vi "AutoRun.vi"() -> ()   [LabVIEW 2016]
uses:
  AutoSteps.ctl
  <vilib>/userdefined/High Color/IMAQdx.ctl
  <vilib>/vision/driver/IMAQdx.llb/IMAQdx Acquisition Mode.ctl
  <vilib>/vision/driver/IMAQdx.llb/IMAQdx Buffer Number Mode.ctl
  <vilib>/vision/driver/NI_Vision_Acquisition_Software.lvlib
panel:
  out "Fitted Circle":T1
  out "ListPoints":dbl[][](array[numeric])
  out "CircleY":dbl
  out "CircleX":dbl
  out "Matches":T2(array[cluster])
  out "形状":enum16{"", "圆形", "三角形", "正方形"}(ring)
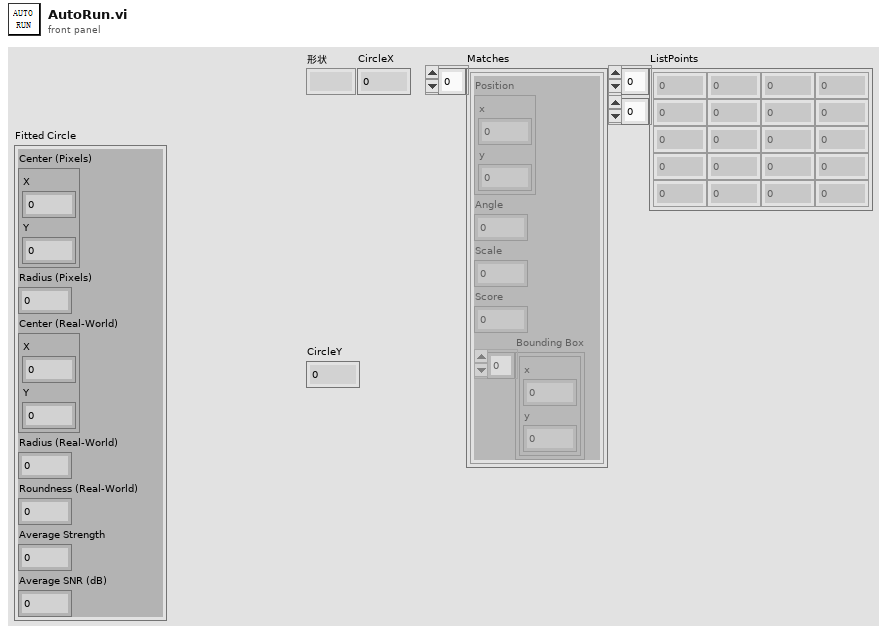
[diagram p1: front panel]
types:
  T1 = cluster{"Center (Pixels)":cluster{"X":sgl, "Y":sgl}, "Radius (Pixels)":dbl, "Center (Real-World)":cluster{"X":sgl, "Y":sgl}, "Radius (Real-World)":dbl, "Roundness (Real-World)":dbl, "Average Strength":dbl, "Average SNR (dB)":dbl}
  T2 = cluster{"Position":cluster{"x":sgl, "y":sgl}, "Angle":sgl, "Scale":sgl, "Score":sgl, "Bounding Box":cluster{"x":sgl, "y":sgl}[]}[]
  T3 = cluster{"Circle":cluster{"CirclePath":path, "Steps":dbl[][], "Points":dbl[][]}, "Trangle":cluster{"TranglePath":path, "Steps":dbl[][], "Points":dbl[][]}, "Square":cluster{"SquarePath":path, "Steps":dbl[][], "Points":dbl[][]}, "Camera":dbl[], "Robot":dbl[]}
  T4 = typedef "AutoSteps.ctl" = enum16{"Nothing", "Initial", "ReadConf", "Wait", "Snap", "ProcePic", "Calculate", "TrancetoPLC", "Error", "Exit"}
  T5 = typedef "IMAQ Image.ctl" = refnum<image>
  T6 = typedef "NI_Vision_Acquisition_Software.lvlib/IMAQdx Acquisition Mode.ctl" = enum32{"One Shot", "Continuous"}
  T7 = typedef "NI_Vision_Acquisition_Software.lvlib/IMAQdx Buffer Number Mode.ctl" = enum32{"Next", "Last", "Buffer Number", "Every", "Last New"}
  T8 = typedef "IMAQdx.ctl" = refnum<k21>
  T9 = cluster{"Position":cluster{"x":sgl, "y":sgl}, "Angle":sgl, "Scale":sgl, "Score":sgl, "Bounding Box":cluster{"x":sgl, "y":sgl}[]}
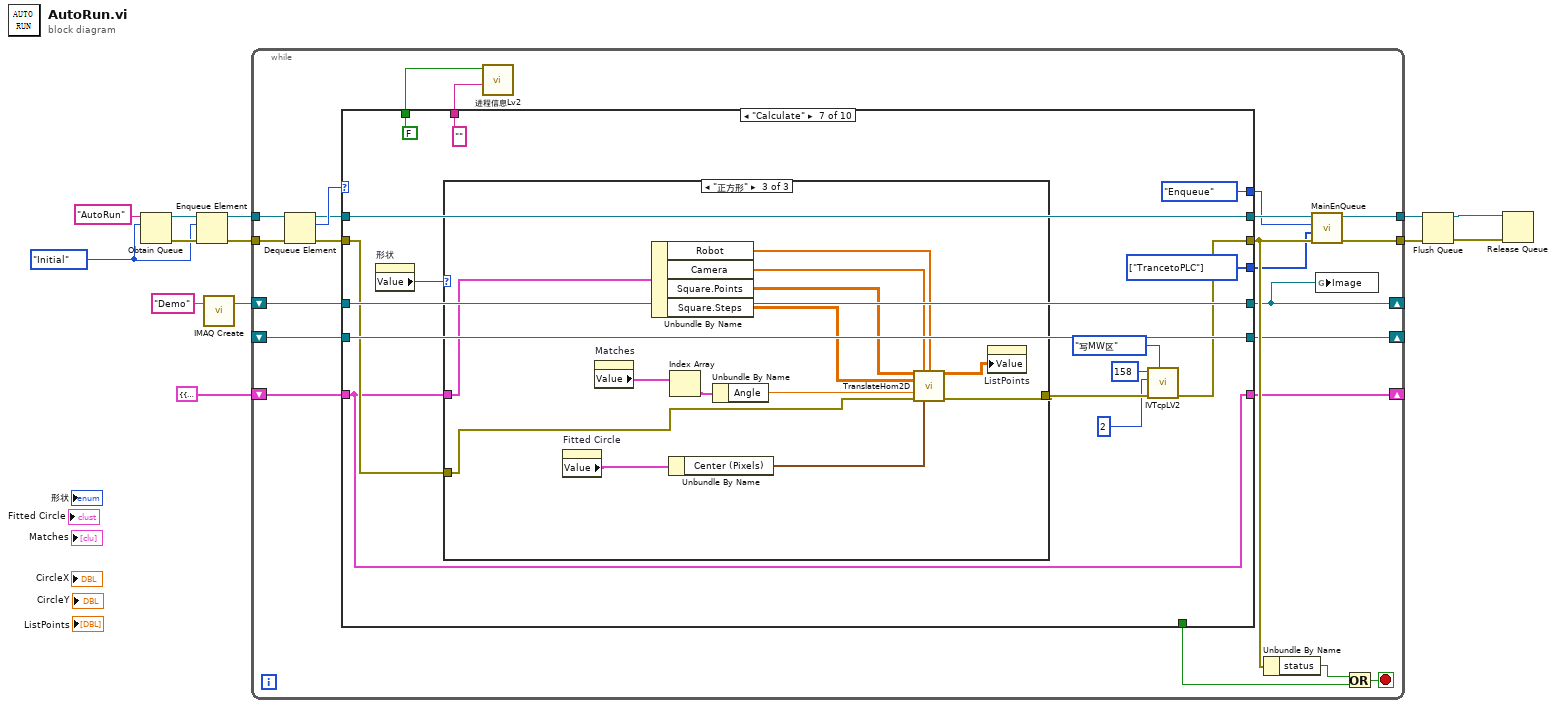
[diagram p0: block diagram]
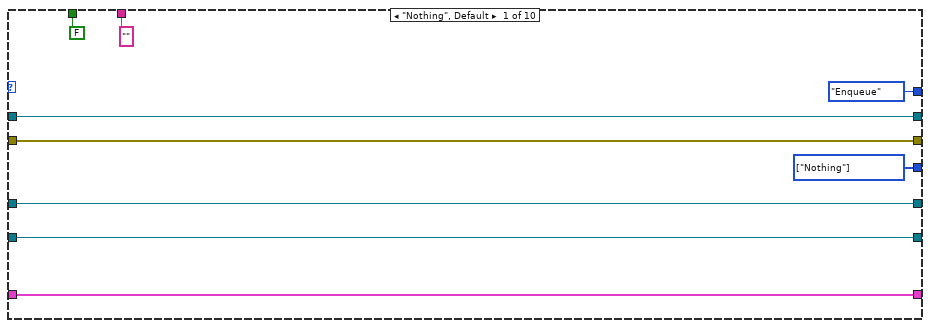
[diagram p2: hidden frame]
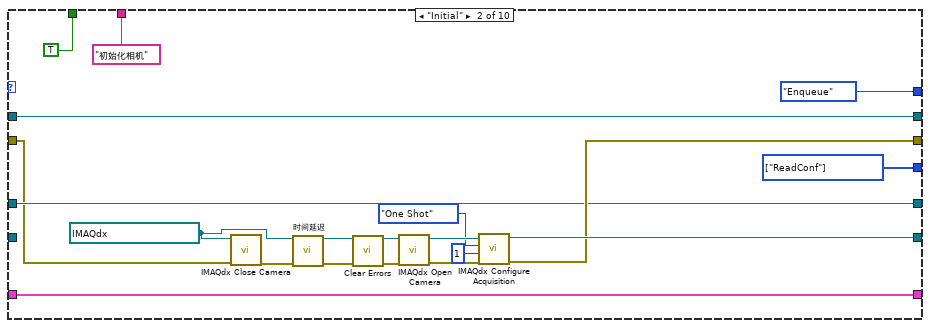
[diagram p3: hidden frame]
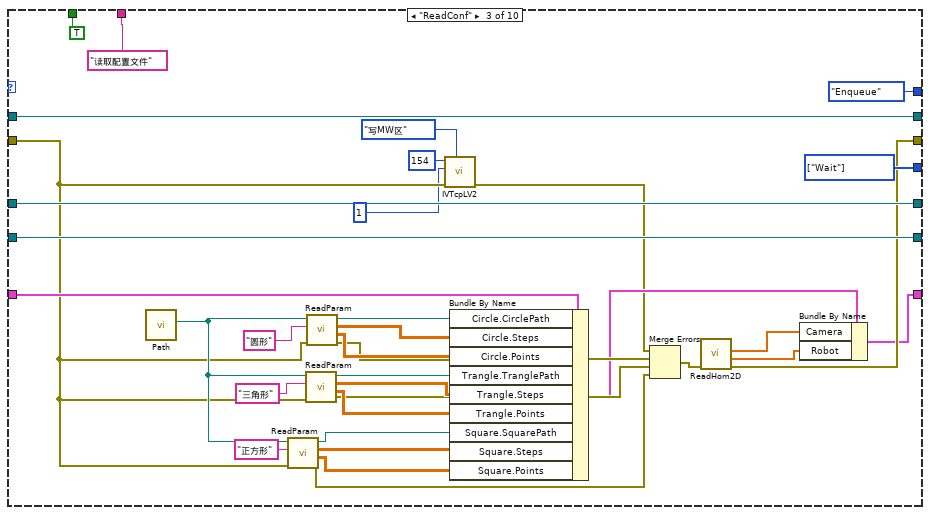
[diagram p4: hidden frame]
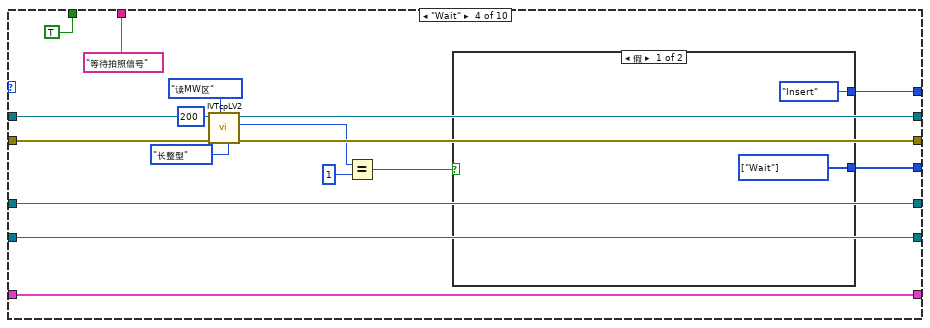
[diagram p5: hidden frame]
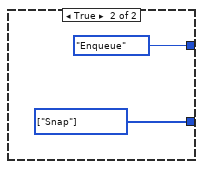
[diagram p6: hidden frame]
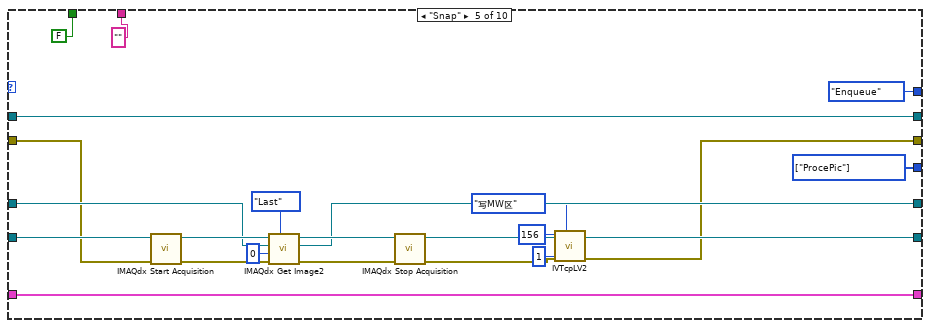
[diagram p7: hidden frame]
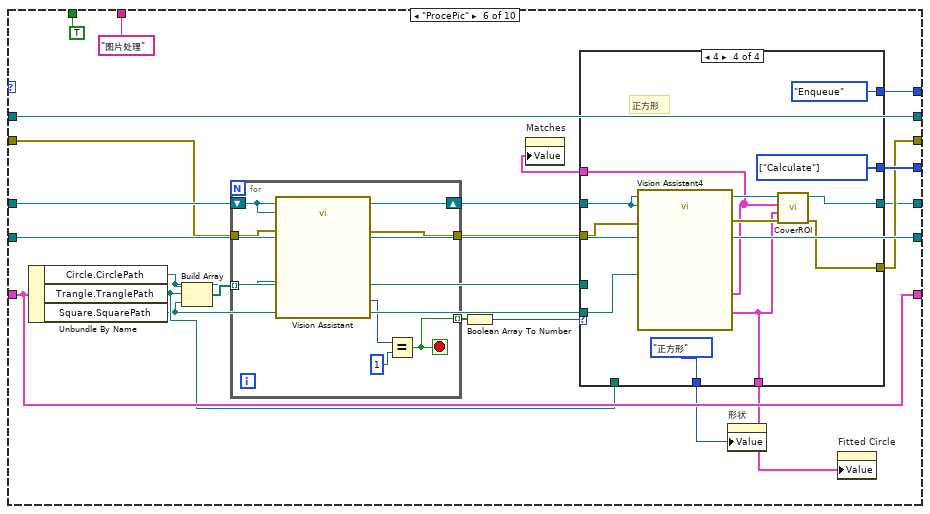
[diagram p8: hidden frame]
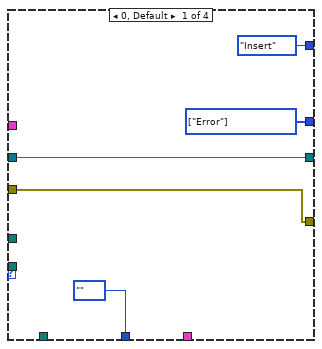
[diagram p9: hidden frame]
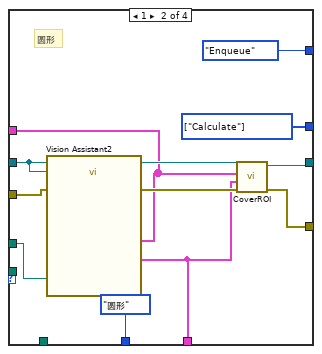
[diagram p10: hidden frame]
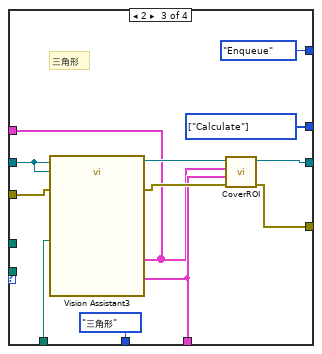
[diagram p11: hidden frame]
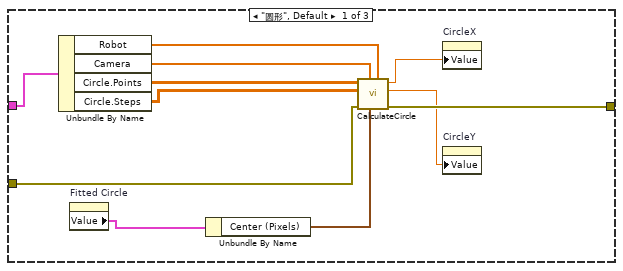
[diagram p12: hidden frame]
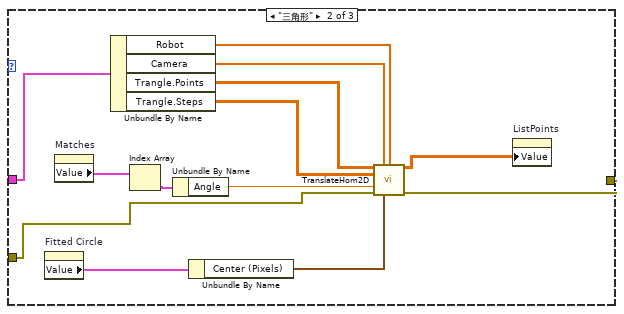
[diagram p13: hidden frame]
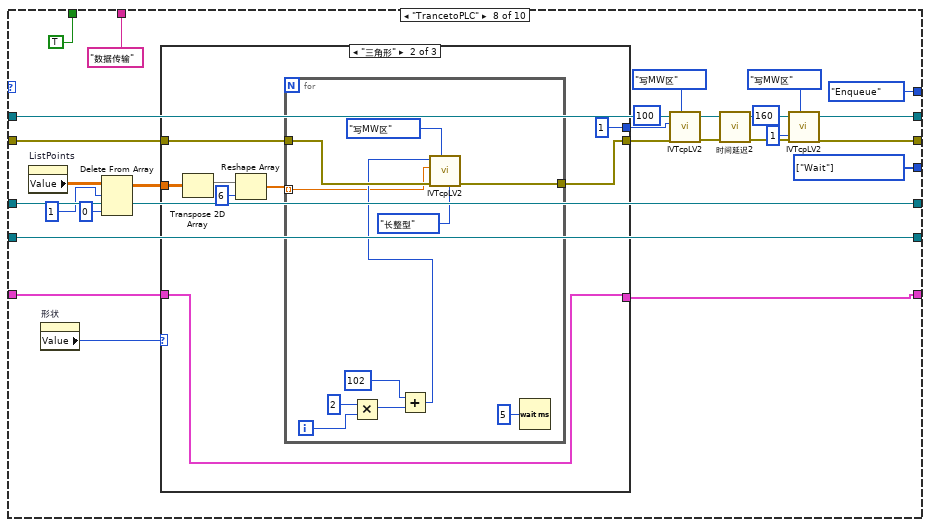
[diagram p14: hidden frame]
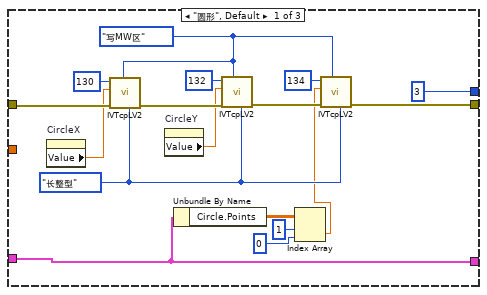
[diagram p15: hidden frame]
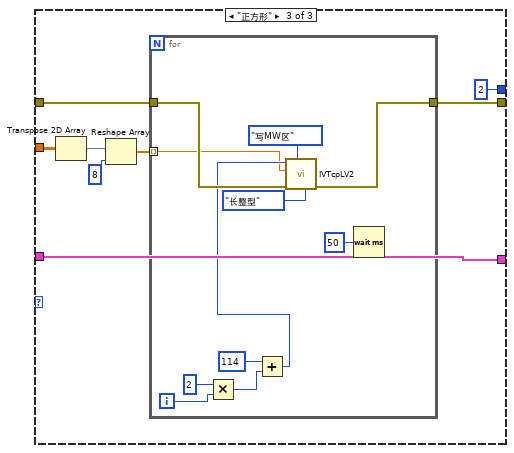
[diagram p16: hidden frame]
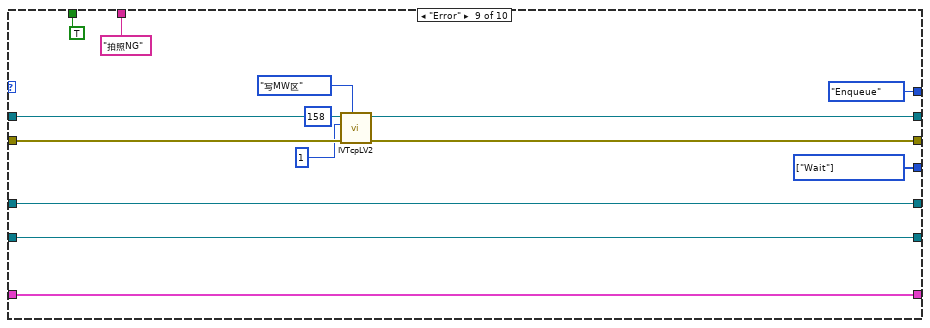
[diagram p17: hidden frame]
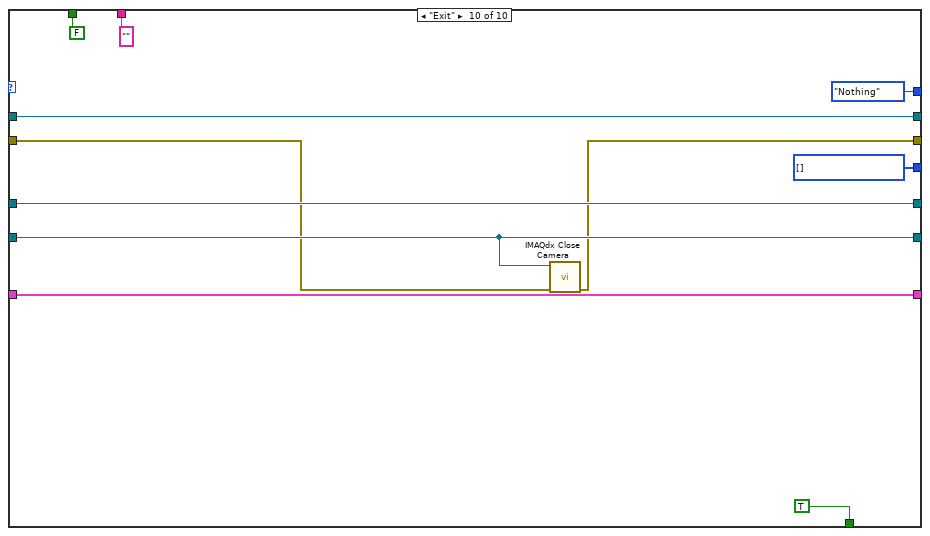
[diagram p18: hidden frame]
diagram:
  w10 = AutoSteps."Initial"
  n1 = Obtain Queue(name (unnamed)="AutoRun" ("名称（未命名）"), element data type=w10) -> (queue out=w12:refnum<queue>, error out=w11:errorcluster)  [unwired: 3 in, 1 out]
  n2 = Enqueue Element(queue=w12, element=w10, error in (no error)=w11) -> (queue out=w9:refnum<queue>, error out=w8:errorcluster)  [unwired: 1 in, 1 out]
  n3 = call "IMAQ Create"("Image Name"="Demo") -> ("New Image"=w2:T5)  [unwired: 4 in, 1 out]
  n4 = while {
    tunnel: w9 -> [w34]
    tunnel: w8 -> [w33]
    tunnel: [w31] -> w7
    tunnel: [w30] -> w4
    shift-right: [w22] -> _
    shift-left: _ -> [w18]
    shift-right: [w21] -> _
    shift-left: w2 -> [w23]
    shift-right: [w16] -> _
    shift-left: T3 {"Circle"={"CirclePath"=path "", "Steps"=[[320.0, 94.0, 0.0], [0.0, 0.0, 0.0], [335.503, 90.501, 0.0]], "Points"=[[35.0]]}, "Trangle"={"TranglePath"=path "", "Steps"=[[320.0, 94.0, 0.0], [0.0, 0.0, 0.0], [335.503, 90.501, 0.0]], "Points"=[[35.0]]}, "Square"={"SquarePath"=path "", "Steps"=[[320.0, 94.0, 0.0], [0.0, 0.0, 0.0], [335.503, 90.501, 0.0]], "Points"=[[35.0]]}, "Camera"=[], "Robot"=[]} -> [w17]
    stop <- w26 stop-if-true
    n5 = Dequeue Element(queue=w34, error in (no error)=w33) -> (queue out=w32:refnum<queue>, element=w35:T4, error out=w29:errorcluster)  [unwired: 1 in, 1 out]
    n6 = case shown="\"Calculate\"" w35 {
      tunnel: w32 -> [w43 w62 w97 w113 w139 w161 w225 w287 w355 w366]
      tunnel: w29 -> [w44 w51 w69 w108 w134 w151 w219 w281 w349 w360]
      tunnel: [w44 w56 w74 w107 w123 w146 w216 w271 w348 w359] -> w27
      tunnel: [w43 w62 w97 w113 w139 w161 w225 w287 w355 w366] -> w28
      tunnel: [_ _ _ _ _ _ _ _ _ TRUE] -> w24
      tunnel: w23 -> [w40 w55 w94 w112 w136 w157 w222 w284 w352 w362]
      tunnel: [w39 w57 w93 w111 w128 w160 w221 w283 w351 w361] -> w22
      tunnel: [w40 w55 w94 w112 w129 w144 w222 w284 w352 w362] -> w21
      tunnel: [enum16{"Nothing", "Insert", "Enqueue"}."Enqueue" ("CMD") enum16{"Nothing", "Insert", "Enqueue"}."Enqueue" ("CMD") enum16{"Nothing", "Insert", "Enqueue"}."Enqueue" ("CMD") w102 enum16{"Nothing", "Insert", "Enqueue"}."Enqueue" ("CMD") w159 enum16{"Nothing", "Insert", "Enqueue"}."Enqueue" ("CMD") enum16{"Nothing", "Insert", "Enqueue"}."Enqueue" ("CMD") enum16{"Nothing", "Insert", "Enqueue"}."Enqueue" ("CMD") enum16{"Nothing", "Insert", "Enqueue"}."Nothing" ("CMD")] -> w20
      tunnel: [w41 w53 w95 w101 w126 w158 w223 w285 w353 w363] -> w19
      tunnel: w18 -> [w39 _ w93 w111 w138 w160 w221 w283 w351 w361]
      tunnel: w17 -> [w38 w52 w88 w100 w125 w155 w218 w276 w350 w358]
      tunnel: [w38 w52 w72 w100 w125 w155 w218 w275 w350 w358] -> w16
      tunnel: [FALSE TRUE TRUE TRUE FALSE TRUE FALSE TRUE TRUE FALSE] -> w15
      tunnel: ["" "初始化相机" "读取配置文件" "等待拍照信号" "" "图片处理" "" "数据传输" "拍照NG" ""] -> w14
      frame "Nothing", Default {
        w41 = T4[] [enum."Nothing"] items=["Nothing", "Initial", "ReadConf", "Wait", "Snap", "ProcePic", "Calculate", "TrancetoPLC", "Error", "Exit"] ("Steps")
      }
      frame "Initial" {
        w53 = T4[] [enum."ReadConf"] items=["Nothing", "Initial", "ReadConf", "Wait", "Snap", "ProcePic", "Calculate", "TrancetoPLC", "Error", "Exit"] ("Steps")
        w50 = T8 "MV-CA060-11GM" ("Session In")
        n7 = call <vilib>:"IMAQdx Close Camera.vi"("error in"=w51, "Session In"=w50) -> ("error out"=w49:errorcluster)  [unwired: 9 in]
        n8 = call "时间延迟"("error in (no error)"=w49) -> ("error out"=w48:errorcluster)  [unwired: 10 in]
        n9 = call <vilib>:"Clear Errors.vi"("error in (no error)"=w48) -> ("error out"=w47:errorcluster)  [unwired: 5 in, 1 out]
        n10 = call <vilib>:"IMAQdx Open Camera.vi"("error in"=w47, "Session In"=w50) -> ("error out"=w60:errorcluster, "Session Out"=w61:T8)  [unwired: 8 in]
        n11 = call <vilib>:"IMAQdx Configure Acquisition.vi"("error in"=w60, "Number of Buffers"=u32 1, "Continuous?"=IMAQdx_Acquisition_Mode."One Shot", "Session In"=w61) -> ("error out"=w56:errorcluster, "Session Out"=w57:T8)  [unwired: 6 in]
      }
      frame "ReadConf" {
        w95 = T4[] [enum."Wait"] items=["Nothing", "Initial", "ReadConf", "Wait", "Snap", "ProcePic", "Calculate", "TrancetoPLC", "Error", "Exit"] ("Steps")
        n12 = call "Path.vi"() -> ("Total"=w89:path)  [unwired: 11 in]
        n13 = call "ReadParam.vi"("error in (no error)"=w69, "机种"="正方形", "路径"=w89) -> ("error out"=w77:errorcluster, "Points"=w79:dbl[][], "Steps"=w80:dbl[][], "TemPath"=w81:path)  [unwired: 5 in]
        n14 = call "ReadParam.vi"("error in (no error)"=w69, "机种"="三角形", "路径"=w89) -> ("error out"=w76:errorcluster, "Points"=w82:dbl[][], "Steps"=w83:dbl[][], "TemPath"=w84:path)  [unwired: 5 in]
        n15 = call "ReadParam.vi"("error in (no error)"=w69, "机种"="圆形", "路径"=w89) -> ("error out"=w78:errorcluster, "Points"=w85:dbl[][], "Steps"=w86:dbl[][], "TemPath"=w87:path)  [unwired: 5 in]
        n16 = call "IVTcpLV2.vi"("TCP操作模式"=enum16{"打开TCP", "读MW区", "写MW区", "关闭TCP"}."写MW区", "错误输入"=w69, "值"=1, "寄存器MD地址"=154) -> ("错误输出"=w65:errorcluster)  [unwired: 4 in, 3 out]
        n17 = Bundle By Name(cluster=w88, "Circle.CirclePath"=w87, "Circle.Steps"=w86, "Circle.Points"=w85, "Trangle.TranglePath"=w84, "Trangle.Steps"=w83, "Trangle.Points"=w82, "Square.SquarePath"=w81, "Square.Steps"=w80, "Square.Points"=w79) -> (w73:T3)
        n18 = Merge Errors(w65, w78, w76, w77) -> (w75:errorcluster)
        n19 = call "ReadHom2D.vi"("error in (no error)"=w75) -> ("error out"=w74:errorcluster, "Robot"=w70:dbl[], "Camera"=w71:dbl[])  [unwired: 7 in, 1 out]
        n20 = Bundle By Name(cluster=w73, "Camera"=w71, "Robot"=w70) -> (w72:T3)
      }
      frame "Wait" {
        n21 = call "IVTcpLV2.vi"("数值类型"=enum16{"长整型", "双精度"}."长整型", "TCP操作模式"=enum16{"打开TCP", "读MW区", "写MW区", "关闭TCP"}."读MW区", "错误输入"=w108, "寄存器MD地址"=200) -> ("错误输出"=w107:errorcluster, "数值"=w105:u32)  [unwired: 4 in, 2 out]
        n22 = Equal?(x=w105, y=u32 1) -> (x = y?=w104:bool)
        n23 = case shown="假" w104 {
          tunnel: [enum16{"Nothing", "Insert", "Enqueue"}."Insert" ("CMD") enum16{"Nothing", "Insert", "Enqueue"}."Enqueue" ("CMD")] -> w102
          tunnel: [w114 w116] -> w101
          frame False {
            w114 = T4[] [enum."Wait"] items=["Nothing", "Initial", "ReadConf", "Wait", "Snap", "ProcePic", "Calculate", "TrancetoPLC", "Error", "Exit"] ("Steps")
          }
          frame True {
            w116 = T4[] [enum."Snap"] items=["Nothing", "Initial", "ReadConf", "Wait", "Snap", "ProcePic", "Calculate", "TrancetoPLC", "Error", "Exit"] ("Steps")
          }
        }
      }
      frame "Snap" {
        w126 = T4[] [enum."ProcePic"] items=["Nothing", "Initial", "ReadConf", "Wait", "Snap", "ProcePic", "Calculate", "TrancetoPLC", "Error", "Exit"] ("Steps")
        n24 = call <vilib>:"IMAQdx Start Acquisition.vi"("error in"=w134, "Session In"=w138) -> ("error out"=w135:errorcluster, "Session Out"=w137:T8)  [unwired: 8 in]
        n25 = call <vilib>:"IMAQdx Get Image2.vi"("Buffer Number Mode (Next)"=IMAQdx_Buffer_Number_Mode."Last", "error in"=w135, "Buffer Number In"=u32 0, "Image In"=w136, "Session In"=w137) -> ("error out"=w132:errorcluster, "Image Out"=w129:T5, "Session Out"=w133:T8)  [unwired: 3 in, 1 out]
        n26 = call <vilib>:"IMAQdx Stop Acquisition.vi"("error in"=w132, "Session In"=w133) -> ("error out"=w124:errorcluster, "Session Out"=w128:T8)  [unwired: 8 in]
        n27 = call "IVTcpLV2.vi"("TCP操作模式"=enum16{"打开TCP", "读MW区", "写MW区", "关闭TCP"}."写MW区", "错误输入"=w124, "值"=1, "寄存器MD地址"=156) -> ("错误输出"=w123:errorcluster)  [unwired: 4 in, 3 out]
      }
      frame "ProcePic" {
        n28 = Unbundle By Name(w155) -> ("Circle.CirclePath"=w147:path, "Trangle.TranglePath"=w141:path, "Square.SquarePath"=w140:path)
        n29 = Build Array(w147, w141, w140) -> (w156:path[])
        n30 = for {
          shift-right: [w209] -> w148
          shift-left: w157 -> [w210]
          tunnel: w156 -> [w208] mode=indexing
          tunnel: [w205] -> w154 mode=indexing
          tunnel: w151 -> [w204]
          tunnel: [w203] -> w145
          stop <- w205 stop-if-true
          n31 = call "Vision Assistant"("Image In"=w210, "Image Dst"=w210, "Template File Path (Pattern Matching 1)"=w208, "error in"=w204) -> ("Image Out"=w209:T5, "Number of Matches (Pattern Matching 1)"=w207:i32, "error out"=w203:errorcluster)  [unwired: 21 in]
          n32 = Equal?(x=w207, y=1) -> (x = y?=w205:bool)
        }
        n33 = Boolean Array To Number(Boolean array=w154) -> (number=w153:u32)
        n34 = case shown="4" w153 {
          tunnel: [enum16{"Nothing", "Insert", "Enqueue"}."Insert" ("CMD") enum16{"Nothing", "Insert", "Enqueue"}."Enqueue" ("CMD") enum16{"Nothing", "Insert", "Enqueue"}."Enqueue" ("CMD") enum16{"Nothing", "Insert", "Enqueue"}."Enqueue" ("CMD")] -> w159
          tunnel: [w165 w177 w189 w201] -> w158
          tunnel: [enum16{"", "圆形", "三角形", "正方形"}."" ("形状") enum16{"", "圆形", "三角形", "正方形"}."圆形" ("形状") enum16{"", "圆形", "三角形", "正方形"}."三角形" ("形状") enum16{"", "圆形", "三角形", "正方形"}."正方形" ("形状")] -> w152
          tunnel: w148 -> [w163 w170 w186 w198]
          tunnel: w147 -> [_ w169 _ _]
          tunnel: [w162 w175 w181 w194] -> w146
          tunnel: w145 -> [w162 w173 w185 w197]
          tunnel: [w163 w171 w183 w196] -> w144
          tunnel: [_ w168 w180 w193] -> w143
          tunnel: [_ w167 w179 w191] -> w142
          tunnel: w141 -> [_ _ w187 _]
          tunnel: w140 -> [_ _ _ w199]
          frame 0, Default {
            w165 = T4[] [enum."Error"] items=["Nothing", "Initial", "ReadConf", "Wait", "Snap", "ProcePic", "Calculate", "TrancetoPLC", "Error", "Exit"] ("Steps")
          }
          frame 1 {
            w177 = T4[] [enum."Calculate"] items=["Nothing", "Initial", "ReadConf", "Wait", "Snap", "ProcePic", "Calculate", "TrancetoPLC", "Error", "Exit"] ("Steps")
            # "圆形"
            n35 = call "Vision Assistant2"("Image In"=w170, "Image Dst"=w170, "Template File Path (Pattern Matching 2)"=w169, "error in"=w173) -> ("Image Out"=w172:T5, "Matches (Pattern Matching 2)"=w167:T2, "Fitted Circle (Find Circular Edge 1)"=w168:T1, "error out"=w174:errorcluster)  [unwired: 20 in]
            n36 = call "CoverROI.vi"("error in (no error)"=w174, "Fitted Circle"=w168, "Matchs"=w167, "Image"=w172) -> ("error out"=w175:errorcluster, "Image Out"=w171:T5)  [unwired: 6 in]
          }
          frame 2 {
            w189 = T4[] [enum."Calculate"] items=["Nothing", "Initial", "ReadConf", "Wait", "Snap", "ProcePic", "Calculate", "TrancetoPLC", "Error", "Exit"] ("Steps")
            # "三角形"
            n37 = call "Vision Assistant3"("Image In"=w186, "Image Dst"=w186, "Template File Path (Pattern Matching 2)"=w187, "error in"=w185) -> ("Image Out"=w184:T5, "Matches (Pattern Matching 2)"=w179:T2, "Fitted Circle (Find Circular Edge 1)"=w180:T1, "error out"=w182:errorcluster)  [unwired: 20 in]
            n38 = call "CoverROI.vi"("error in (no error)"=w182, "Fitted Circle"=w180, "Matchs"=w179, "Image"=w184) -> ("error out"=w181:errorcluster, "Image Out"=w183:T5)  [unwired: 6 in]
          }
          frame 4 {
            w201 = T4[] [enum."Calculate"] items=["Nothing", "Initial", "ReadConf", "Wait", "Snap", "ProcePic", "Calculate", "TrancetoPLC", "Error", "Exit"] ("Steps")
            # "正方形"
            n39 = call "Vision Assistant4"("Image In"=w198, "Image Dst"=w198, "Template File Path (Pattern Matching 2)"=w199, "error in"=w197) -> ("Image Out"=w192:T5, "Matches (Pattern Matching 2)"=w191:T2, "Fitted Circle (Find Circular Edge 1)"=w193:T1, "error out"=w195:errorcluster)  [unwired: 20 in]
            n40 = call "CoverROI.vi"("error in (no error)"=w195, "Fitted Circle"=w193, "Matchs"=w191, "Image"=w192) -> ("error out"=w194:errorcluster, "Image Out"=w196:T5)  [unwired: 6 in]
          }
        }
        n41 = property on="Matches" class="Arr (严格)"("Value"=w142) -> ()  [unwired: 2 in, 2 out]
        n42 = property on="形状" class="Enum (严格)"("Value"=w152) -> ()  [unwired: 2 in, 2 out]
        n43 = property on="Fitted Circle" class="Clust (严格)"("Value"=w143) -> ()  [unwired: 2 in, 2 out]
      }
      frame "Calculate" {
        w223 = T4[] [enum."TrancetoPLC"] items=["Nothing", "Initial", "ReadConf", "Wait", "Snap", "ProcePic", "Calculate", "TrancetoPLC", "Error", "Exit"] ("Steps")
        n44 = property on="形状" class="Enum (严格)"() -> ("Value"=w220:enum16{"", "圆形", "三角形", "正方形"})  [unwired: 2 in, 2 out]
        n45 = case shown="\"正方形\"" w220 {
          tunnel: w218 -> [w236 w249 w254]
          tunnel: [w233 w239 w252] -> w217
          tunnel: w219 -> [w232 w240 w253]
          frame "圆形", Default {
            n46 = Unbundle By Name(w236) -> ("Robot"=w235:dbl[], "Camera"=w234:dbl[], "Circle.Points"=w228:dbl[][], "Circle.Steps"=w227:dbl[][])
            n47 = property on="Fitted Circle" class="Clust (严格)"() -> ("Value"=w226:T1)  [unwired: 2 in, 2 out]
            n48 = Unbundle By Name(w226) -> ("Center (Pixels)"=w229:cluster{"X":sgl, "Y":sgl})
            n49 = call "CalculateCircle.vi"("Robot"=w235, "RealCamera"=w229, "Camera"=w234, "错误输入（无错误）"=w232, "Circle.Steps"=w227, "Circle.Points"=w228) -> ("错误输出"=w233:errorcluster, "RobotY"=w230:dbl, "RobotX"=w231:dbl)  [unwired: 3 in]
            n50 = property on="CircleX" class="DigNum (严格)"("Value"=w231) -> ()  [unwired: 2 in, 2 out]
            n51 = property on="CircleY" class="DigNum (严格)"("Value"=w230) -> ()  [unwired: 2 in, 2 out]
          }
          frame "三角形" {
            n52 = property on="Fitted Circle" class="Clust (严格)"() -> ("Value"=w237:T1)  [unwired: 2 in, 2 out]
            n53 = property on="Matches" class="Arr (严格)"() -> ("Value"=w244:T2)  [unwired: 2 in, 2 out]
            n54 = Unbundle By Name(w249) -> ("Robot"=w248:dbl[], "Camera"=w247:dbl[], "Trangle.Points"=w246:dbl[][], "Trangle.Steps"=w245:dbl[][])
            n55 = Index Array(array=w244) -> (element=w243:T9)  [unwired: 1 in]
            n56 = Unbundle By Name(w243) -> ("Angle"=w242:sgl)
            n57 = Unbundle By Name(w237) -> ("Center (Pixels)"=w241:cluster{"X":sgl, "Y":sgl})
            n58 = call "TranslateHom2D.vi"("points"=w246, "Camera"=w247, "Robot"=w248, "Steps"=w245, "Angle"=w242, "错误输入（无错误）"=w240, "RealCamera"=w241) -> ("ListPoints"=w238:dbl[][], "错误输出"=w239:errorcluster)  [unwired: 6 in, 1 out]
            n59 = property on="ListPoints" class="Arr (严格)"("Value"=w238) -> ()  [unwired: 2 in, 2 out]
          }
          frame "正方形" {
            n60 = property on="Fitted Circle" class="Clust (严格)"() -> ("Value"=w250:T1)  [unwired: 2 in, 2 out]
            n61 = property on="Matches" class="Arr (严格)"() -> ("Value"=w258:T2)  [unwired: 2 in, 2 out]
            n62 = Unbundle By Name(w254) -> ("Robot"=w262:dbl[], "Camera"=w261:dbl[], "Square.Points"=w260:dbl[][], "Square.Steps"=w259:dbl[][])
            n63 = Unbundle By Name(w250) -> ("Center (Pixels)"=w255:cluster{"X":sgl, "Y":sgl})
            n64 = Index Array(array=w258) -> (element=w257:T9)  [unwired: 1 in]
            n65 = Unbundle By Name(w257) -> ("Angle"=w256:sgl)
            n66 = call "TranslateHom2D.vi"("points"=w260, "Camera"=w261, "Robot"=w262, "Steps"=w259, "Angle"=w256, "错误输入（无错误）"=w253, "RealCamera"=w255) -> ("ListPoints"=w251:dbl[][], "错误输出"=w252:errorcluster)  [unwired: 6 in, 1 out]
            n67 = property on="ListPoints" class="Arr (严格)"("Value"=w251) -> ()  [unwired: 2 in, 2 out]
          }
        }
        n68 = call "IVTcpLV2.vi"("TCP操作模式"=enum16{"打开TCP", "读MW区", "写MW区", "关闭TCP"}."写MW区", "错误输入"=w217, "值"=2, "寄存器MD地址"=158) -> ("错误输出"=w216:errorcluster)  [unwired: 4 in, 3 out]
      }
      frame "TrancetoPLC" {
        w285 = T4[] [enum."Wait"] items=["Nothing", "Initial", "ReadConf", "Wait", "Snap", "ProcePic", "Calculate", "TrancetoPLC", "Error", "Exit"] ("Steps")
        n69 = property on="ListPoints" class="Arr (严格)"() -> ("Value"=w274:dbl[][])  [unwired: 2 in, 2 out]
        n70 = property on="形状" class="Enum (严格)"() -> ("Value"=w282:enum16{"", "圆形", "三角形", "正方形"})  [unwired: 2 in, 2 out]
        n71 = Delete From Array(array=w274, length=1 ("长度"), index (col)=0 ("索引 (行)")) -> (array with subset deleted=w272:dbl[][])  [unwired: 1 in, 1 out]
        n72 = case shown="\"三角形\"" w282 {
          tunnel: w281 -> [w303 w310 w328]
          tunnel: [w297 w309 w327] -> w280
          tunnel: [3 1 2] -> w277
          tunnel: w276 -> [w294 w311 w326]
          tunnel: [w294 w311 w326] -> w275
          tunnel: w272 -> [_ w308 w325]
          frame "圆形", Default {
            w295 = enum16{"长整型", "双精度"}."长整型" ("数值类型")
            w296 = enum16{"打开TCP", "读MW区", "写MW区", "关闭TCP"}."写MW区" ("TCP操作模式")
            n73 = property on="CircleX" class="DigNum (严格)"() -> ("Value"=w290:dbl)  [unwired: 2 in, 2 out]
            n74 = call "IVTcpLV2.vi"("数值类型"=w295, "TCP操作模式"=w296, "错误输入"=w303, "值"=w290, "寄存器MD地址"=130) -> ("错误输出"=w302:errorcluster)  [unwired: 3 in, 3 out]
            n75 = property on="CircleY" class="DigNum (严格)"() -> ("Value"=w289:dbl)  [unwired: 2 in, 2 out]
            n76 = Unbundle By Name(w294) -> ("Circle.Points"=w293:dbl[][])
            n77 = call "IVTcpLV2.vi"("数值类型"=w295, "TCP操作模式"=w296, "错误输入"=w302, "值"=w289, "寄存器MD地址"=132) -> ("错误输出"=w298:errorcluster)  [unwired: 3 in, 3 out]
            n78 = Index Array(array=w293, index (row)=1 ("索引 (行)"), index (col)=0 ("索引 (行)")) -> (element=w288:dbl)
            n79 = call "IVTcpLV2.vi"("数值类型"=w295, "TCP操作模式"=w296, "错误输入"=w298, "值"=w288, "寄存器MD地址"=134) -> ("错误输出"=w297:errorcluster)  [unwired: 3 in, 3 out]
          }
          frame "三角形" {
            n80 = Transpose 2D Array(2D array=w308) -> (transposed array=w307:dbl[][])
            n81 = Reshape Array(w307, 6 ("维数大小")) -> (w305:dbl[])
            n82 = for {
              tunnel: w305 -> [w316] mode=indexing
              tunnel: w310 -> [w323]
              tunnel: [w313] -> w309
              i -> [w314]
              n83 = Multiply(x=2, y=w314) -> (x*y=w319:i32)
              n84 = Add(x=102, y=w319) -> (x+y=w317:i32)
              n85 = call "IVTcpLV2.vi"("数值类型"=enum16{"长整型", "双精度"}."长整型", "TCP操作模式"=enum16{"打开TCP", "读MW区", "写MW区", "关闭TCP"}."写MW区", "错误输入"=w323, "值"=w316, "寄存器MD地址"=w317) -> ("错误输出"=w313:errorcluster)  [unwired: 3 in, 3 out]
              n86 = Wait (ms)(milliseconds to wait=u32 5 ("等待时间（毫秒）")) -> ()  [unwired: 1 out]
            }
          }
          frame "正方形" {
            n87 = Transpose 2D Array(2D array=w325) -> (transposed array=w324:dbl[][])
            n88 = Reshape Array(w324, 8 ("维数大小")) -> (w329:dbl[])
            n89 = for {
              tunnel: w329 -> [w333] mode=indexing
              tunnel: w328 -> [w342]
              tunnel: [w334] -> w327
              i -> [w339]
              n90 = Multiply(x=2, y=w339) -> (x*y=w337:i32)
              n91 = Add(x=114, y=w337) -> (x+y=w336:i32)
              n92 = call "IVTcpLV2.vi"("数值类型"=enum16{"长整型", "双精度"}."长整型", "TCP操作模式"=enum16{"打开TCP", "读MW区", "写MW区", "关闭TCP"}."写MW区", "错误输入"=w342, "值"=w333, "寄存器MD地址"=w336) -> ("错误输出"=w334:errorcluster)  [unwired: 3 in, 3 out]
              n93 = Wait (ms)(milliseconds to wait=u32 50 ("等待时间（毫秒）")) -> ()  [unwired: 1 out]
            }
          }
        }
        n94 = call "IVTcpLV2.vi"("TCP操作模式"=enum16{"打开TCP", "读MW区", "写MW区", "关闭TCP"}."写MW区", "错误输入"=w280, "值"=w277, "寄存器MD地址"=100) -> ("错误输出"=w267:errorcluster)  [unwired: 4 in, 3 out]
        n95 = call "时间延迟2"("error in (no error)"=w267) -> ("error out"=w266:errorcluster)  [unwired: 10 in]
        n96 = call "IVTcpLV2.vi"("TCP操作模式"=enum16{"打开TCP", "读MW区", "写MW区", "关闭TCP"}."写MW区", "错误输入"=w266, "值"=1, "寄存器MD地址"=160) -> ("错误输出"=w271:errorcluster)  [unwired: 4 in, 3 out]
      }
      frame "Error" {
        w353 = T4[] [enum."Wait"] items=["Nothing", "Initial", "ReadConf", "Wait", "Snap", "ProcePic", "Calculate", "TrancetoPLC", "Error", "Exit"] ("Steps")
        n97 = call "IVTcpLV2.vi"("TCP操作模式"=enum16{"打开TCP", "读MW区", "写MW区", "关闭TCP"}."写MW区", "错误输入"=w349, "值"=1, "寄存器MD地址"=158) -> ("错误输出"=w348:errorcluster)  [unwired: 4 in, 3 out]
      }
      frame "Exit" {
        w363 = T4[] [] items=["Nothing", "Initial", "ReadConf", "Wait", "Snap", "ProcePic", "Calculate", "TrancetoPLC", "Error", "Exit"] ("Steps")
        n98 = call <vilib>:"IMAQdx Close Camera.vi"("error in"=w360, "Session In"=w361) -> ("error out"=w359:errorcluster)  [unwired: 9 in]
      }
    }
    n99 = call "进程信息Lv2.vi"("状态"=w14, "显示？"=w15) -> ()  [unwired: 5 in, 1 out]
    n100 = Unbundle By Name(w27) -> ("status"=w25:bool)
    n101 = call "MainEnQueue.vi"("错误输入（无错误）"=w27, "Steps"=w19, "CMD"=w20, "队列输入"=w28) -> ("error out"=w30:errorcluster, "队列输出"=w31:refnum<queue>)  [unwired: 6 in]
    n102 = global write "全局.vi" "Image"(w21) -> ()
    n103 = Or(x=w25, y=w24) -> (x .or. y?=w26:bool)
  }
  n104 = Flush Queue(queue=w7, error in (no error)=w4) -> (queue out=w5:refnum<queue>, error out=w6:errorcluster)  [unwired: 1 out]
  n105 = Release Queue(queue=w5, error in (no error)=w6) -> ()  [unwired: 1 in, 3 out]
